vi "Timed motor direction switch.vi"() -> ()   [LabVIEW 2015]
panel:
  out "GREEN = PASS 2":bool caption="Passed"
  out "Sheath Forward":dynamicdata(graph) caption="Tested Signals"
  out "Guide Backward":dynamicdata(graph) caption="Tested Signals"
  out "Guide Forward":dynamicdata(graph) caption="Tested Signals"
  out "XY Graph":cluster{"X":dbl, "Y":dbl}[](graph)
  out "Encoder Graph":waveform(dbl)(graph)
  in  "Sensei":bool
  in  "Boolean 10":bool
  in  "Boolean 9":bool
  in  "Boolean 8":bool
  in  "Boolean 7":bool
  in  "Boolean 6":bool
  in  "Boolean 5":bool
  in  "Boolean 4":bool
  in  "Boolean 3":bool
  out "GREEN = PASS":bool caption="Passed"
  out "Sheath Forward":dynamicdata(graph) caption="Tested Signals"
  out "V v. t (2nd)":cluster{"X":dbl, "Y":dbl}[](graph)
  out "T v. t (2nd)":cluster{"X":dbl, "Y":dbl}[](graph)
  out "V v. t (1st)":cluster{"X":dbl, "Y":dbl}[](graph)
  out "T v. t (1st)":cluster{"X":dbl, "Y":dbl}[](graph)
  in  "TORQUE SET POINT":dbl caption="Torque setpoint"
  # "SELECT MOTOR AND PRESS RUN"
  # "SELECT ONE MOTOR AT A TIME"
  # "Guide Carriage"
  # "Sheath Carriage"
  # "Magellan"
  # "3\n7"
  # "X\n2"
  # "6\n3"
  # "2\n8"
  # "X\n1"
  # "4\n9"
  # "7\n4"
  # "1\n6"
  # "FORWARD ROTATION"
  # "BACKWARD ROTATION"
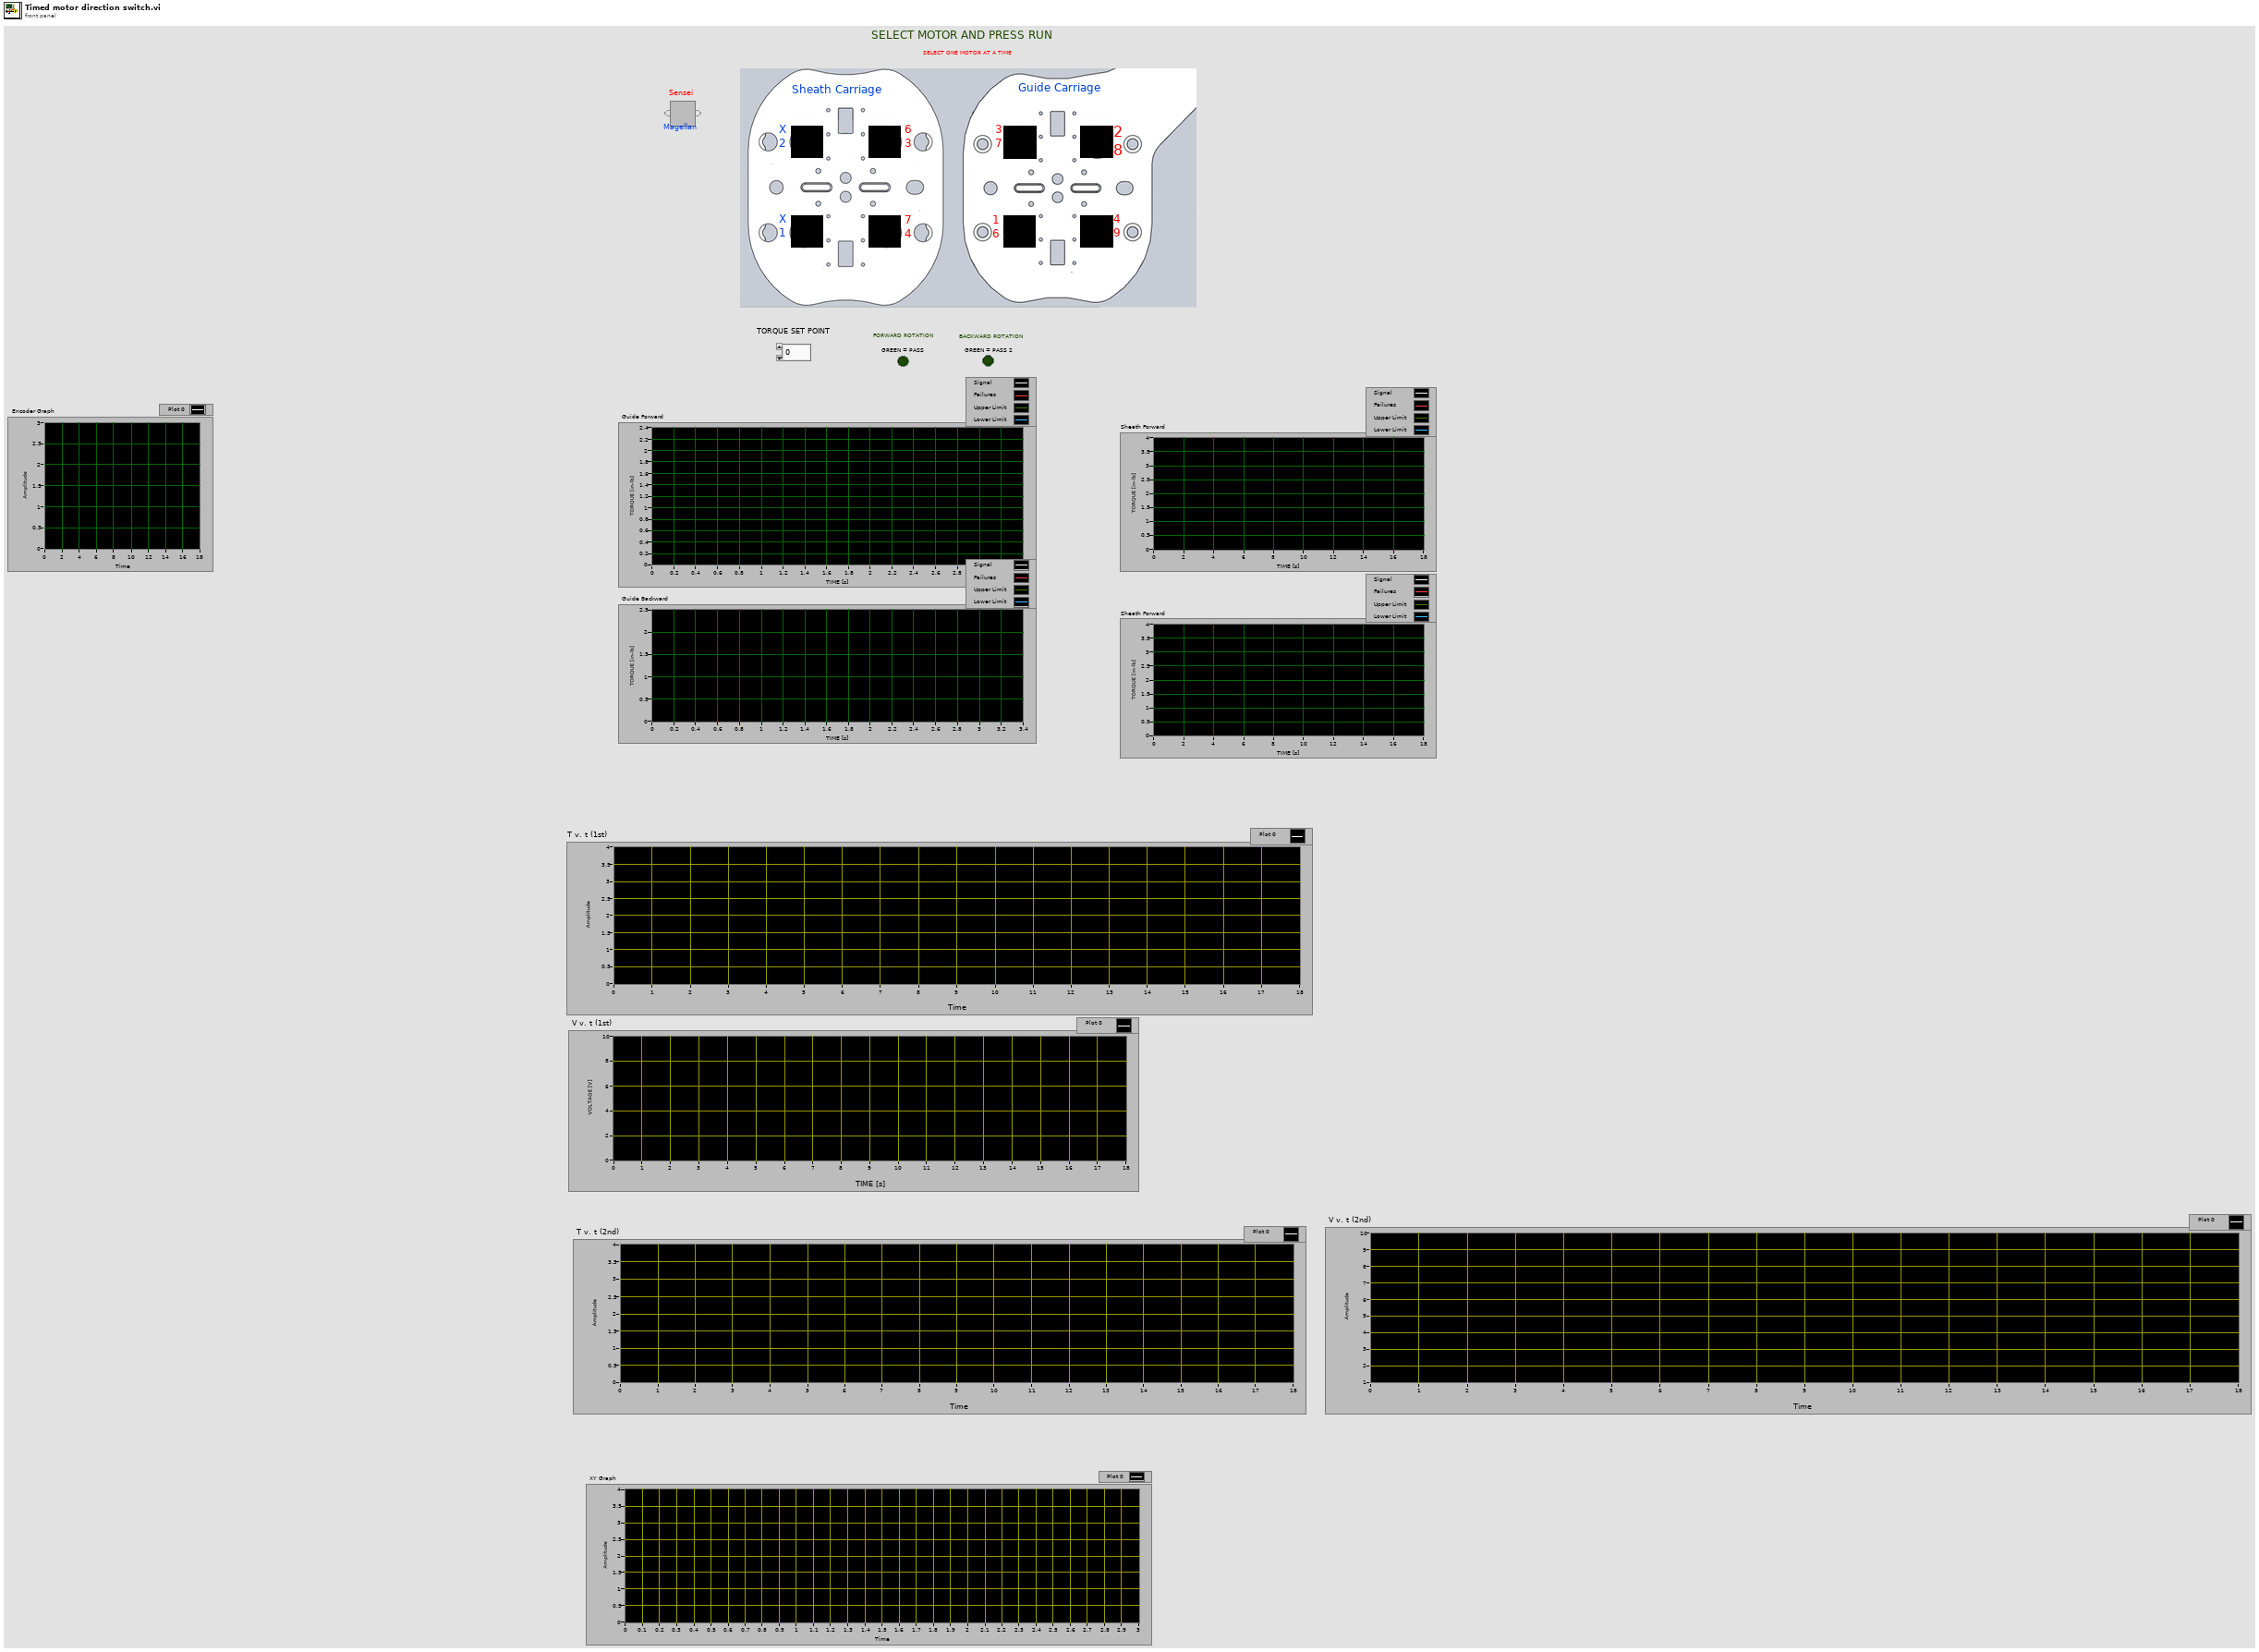
[diagram p1: front panel]
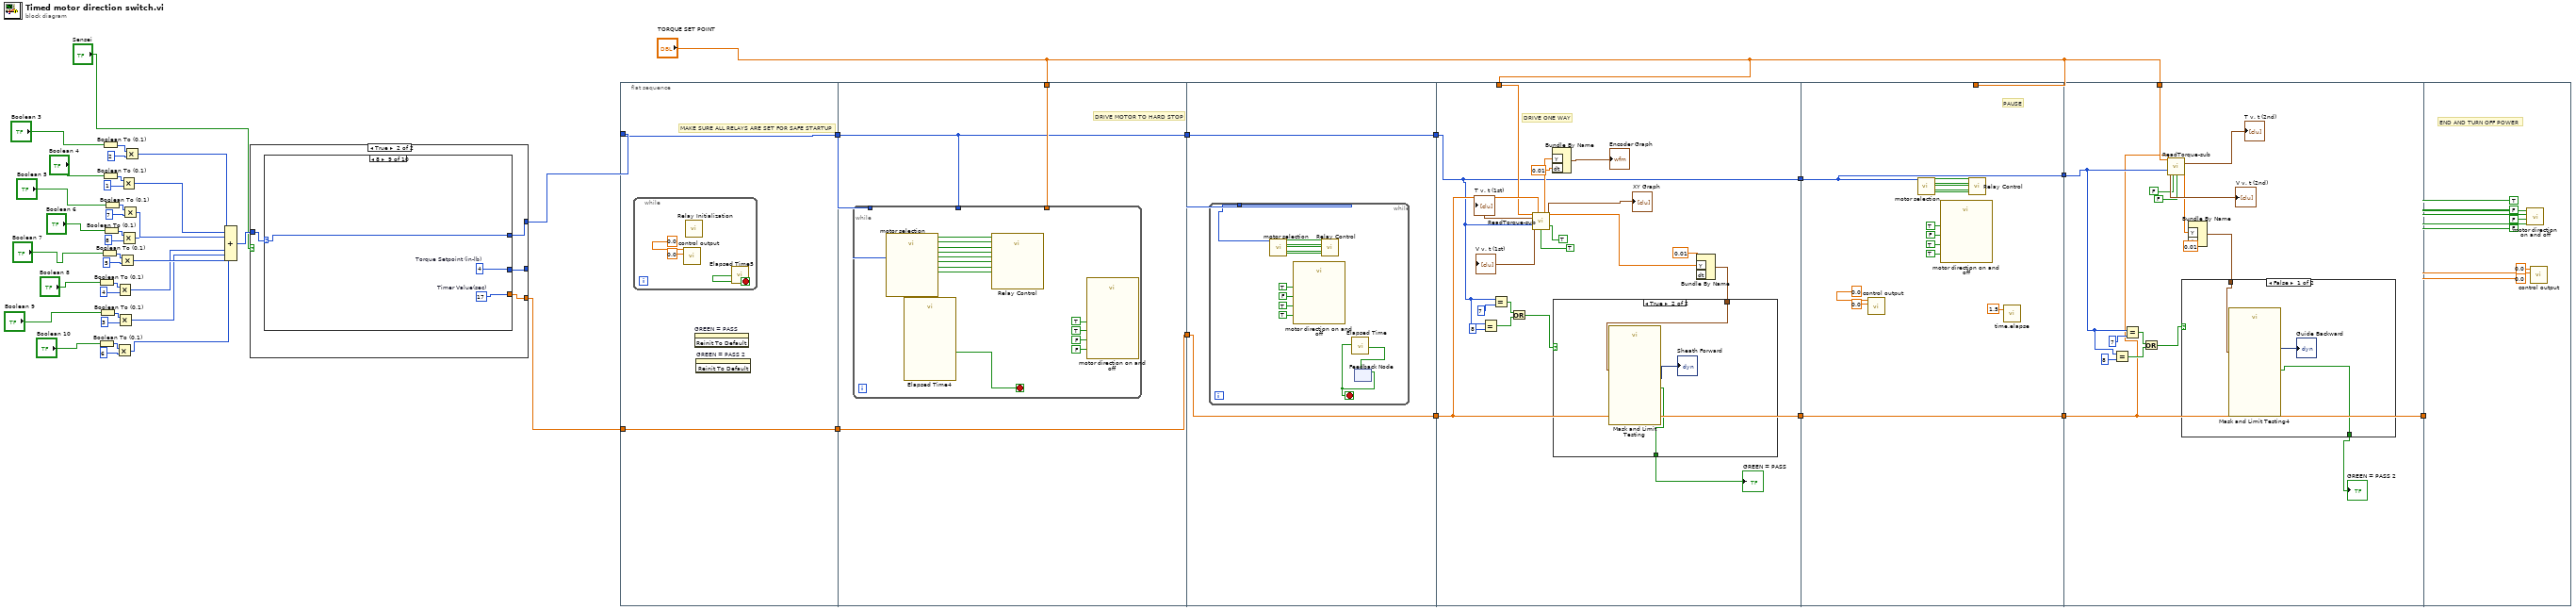
[diagram p0: block diagram]
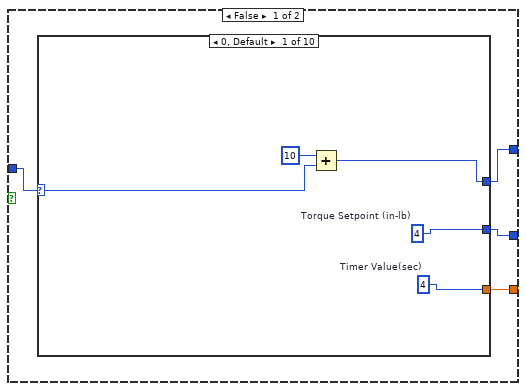
[diagram p2: hidden frame]
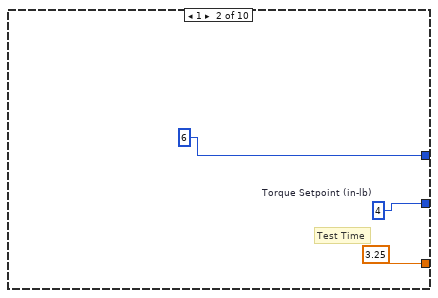
[diagram p3: hidden frame]
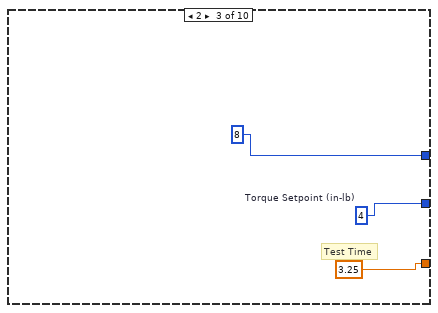
[diagram p4: hidden frame]
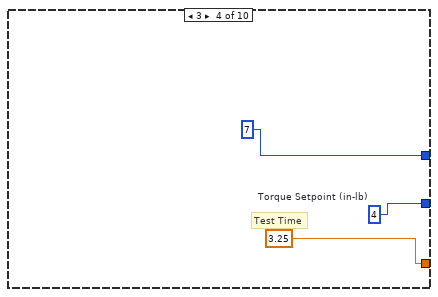
[diagram p5: hidden frame]
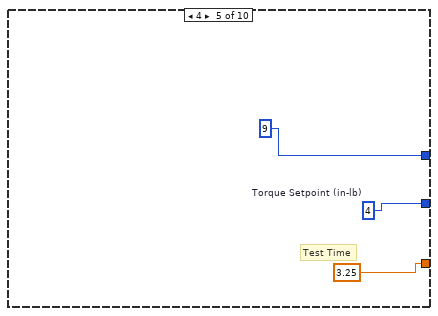
[diagram p6: hidden frame]
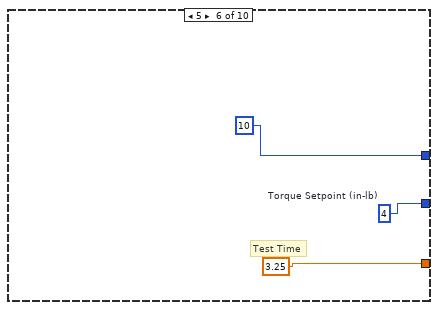
[diagram p7: hidden frame]
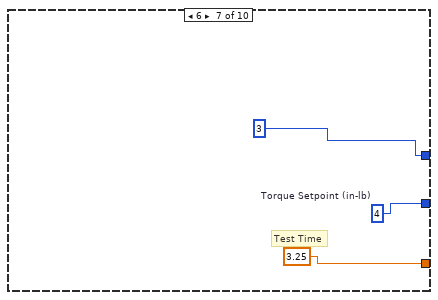
[diagram p8: hidden frame]
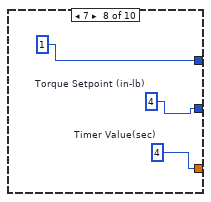
[diagram p9: hidden frame]
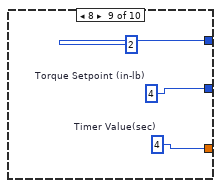
[diagram p10: hidden frame]
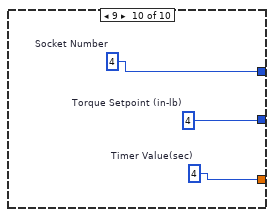
[diagram p11: hidden frame]
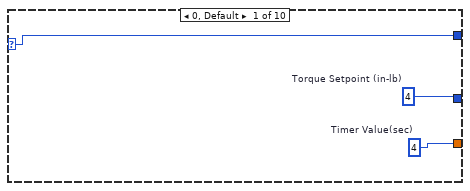
[diagram p12: hidden frame]
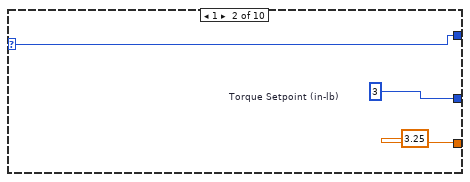
[diagram p13: hidden frame]
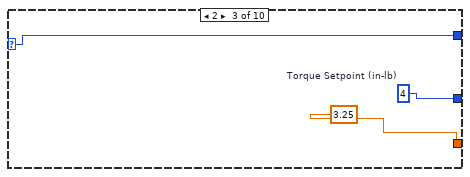
[diagram p14: hidden frame]
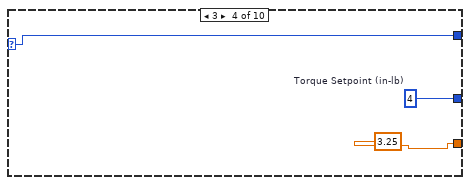
[diagram p15: hidden frame]
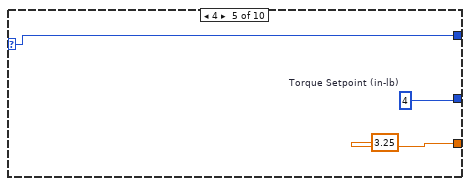
[diagram p16: hidden frame]
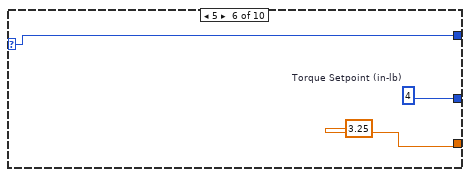
[diagram p17: hidden frame]
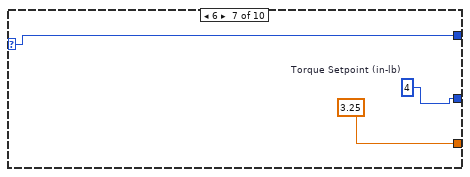
[diagram p18: hidden frame]
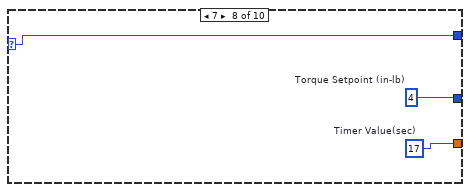
[diagram p19: hidden frame]
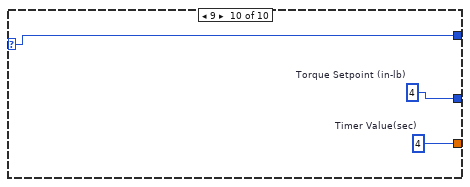
[diagram p20: hidden frame]
diagram:
  n1 = Boolean To (0,1)(Boolean="Boolean 10") -> (0, 1=w28:i16)
  n2 = Boolean To (0,1)(Boolean="Boolean 8") -> (0, 1=w32:i16)
  n3 = Boolean To (0,1)(Boolean="Boolean 9") -> (0, 1=w30:i16)
  n4 = Boolean To (0,1)(Boolean="Boolean 7") -> (0, 1=w34:i16)
  n5 = Boolean To (0,1)(Boolean="Boolean 3") -> (0, 1=w42:i16)
  n6 = Boolean To (0,1)(Boolean="Boolean 4") -> (0, 1=w40:i16)
  n7 = Boolean To (0,1)(Boolean="Boolean 6") -> (0, 1=w36:i16)
  n8 = Boolean To (0,1)(Boolean="Boolean 5") -> (0, 1=w38:i16)
  n9 = Multiply(x=w28, y=i16 6) -> (x*y=w19:i16)
  n10 = Multiply(x=w32, y=i16 4) -> (x*y=w21:i16)
  n11 = Multiply(x=w30, y=i16 3) -> (x*y=w20:i16)
  n12 = Multiply(x=w34, y=i16 5) -> (x*y=w22:i16)
  n13 = Multiply(x=w40, y=i16 1) -> (x*y=w25:i16)
  n14 = Multiply(x=w36, y=i16 8) -> (x*y=w23:i16)
  n15 = Multiply(x=w38, y=i16 7) -> (x*y=w24:i16)
  n16 = Multiply(x=w42, y=i16 2) -> (x*y=w26:i16)
  n17 = Compound Arithmetic op=ADD(w26, w25, w24, w23, w22, w21, w20, w19) -> (w18:i16)
  n18 = case shown="True" "Sensei" {
    tunnel: [w52 w88] -> w8
    tunnel: w18 -> [w51 w87]
    tunnel: [w50 w85] -> w6
    tunnel: [w49 w86] -> _
    frame False {
      n19 = case shown="0, Default" w51 {
        selector: w51 -> [w55 _ _ _ _ _ _ _ _ _]
        tunnel: [w56 6 ("x") 8 ("x") 7 ("x") 9 ("x") 10 ("x") 3 ("x") 1 ("x") 2 ("x") w84] -> w52
        tunnel: [w54 w59 w62 w65 w68 w71 w74 w77 w80 w83] -> w49
        tunnel: [w53 3.25 3.25 3.25 3.25 3.25 3.25 w76 w79 w82] -> w50
        frame 0, Default {
          w53 = 4  # Timer Value(sec)
          w54 = 4  # Torque Setpoint (in-lb)
          n20 = Add(x=10, y=w55) -> (x+y=w56:i32)
        }
        frame 1 {
          w59 = 4  # Torque Setpoint (in-lb)
          # "Test Time"
        }
        frame 2 {
          w62 = 4  # Torque Setpoint (in-lb)
          # "Test Time"
        }
        frame 3 {
          w65 = 4  # Torque Setpoint (in-lb)
          # "Test Time"
        }
        frame 4 {
          w68 = 4  # Torque Setpoint (in-lb)
          # "Test Time"
        }
        frame 5 {
          w71 = 4  # Torque Setpoint (in-lb)
          # "Test Time"
        }
        frame 6 {
          w74 = 4  # Torque Setpoint (in-lb)
          # "Test Time"
        }
        frame 7 {
          w76 = 4  # Timer Value(sec)
          w77 = 4  # Torque Setpoint (in-lb)
        }
        frame 8 {
          w79 = 4  # Timer Value(sec)
          w80 = 4  # Torque Setpoint (in-lb)
        }
        frame 9 {
          w82 = 4  # Timer Value(sec)
          w83 = 4  # Torque Setpoint (in-lb)
          w84 = 4  # Socket Number
        }
      }
    }
    frame True {
      n21 = case shown="8" w87 {
        selector: w87 -> [w91 w94 w97 w100 w103 w106 w109 w112 w115 w118]
        tunnel: [w91 w94 w97 w100 w103 w106 w109 w112 w115 w118] -> w88
        tunnel: [w90 w93 w96 w99 w102 w105 w108 w111 w114 w117] -> w86
        tunnel: [w89 3.25 3.25 3.25 3.25 3.25 3.25 w110 w113 w116] -> w85
        frame 0, Default {
          w89 = 4  # Timer Value(sec)
          w90 = 4  # Torque Setpoint (in-lb)
        }
        frame 1 {
          w93 = 3  # Torque Setpoint (in-lb)
        }
        frame 2 {
          w96 = 4  # Torque Setpoint (in-lb)
        }
        frame 3 {
          w99 = 4  # Torque Setpoint (in-lb)
        }
        frame 4 {
          w102 = 4  # Torque Setpoint (in-lb)
        }
        frame 5 {
          w105 = 4  # Torque Setpoint (in-lb)
        }
        frame 6 {
          w108 = 4  # Torque Setpoint (in-lb)
        }
        frame 7 {
          w110 = 17  # Timer Value(sec)
          w111 = 4  # Torque Setpoint (in-lb)
        }
        frame 8 {
          w113 = 17  # Timer Value(sec)
          w114 = 4  # Torque Setpoint (in-lb)
        }
        frame 9 {
          w116 = 4  # Timer Value(sec)
          w117 = 4  # Torque Setpoint (in-lb)
        }
      }
    }
  }
  n22 = flat-sequence {
    tunnel: w8 -> [w120]
    tunnel: [w120] -> w48
    tunnel: w6 -> [w119]
    tunnel: [w119] -> w5
    tunnel: w48 -> [w125]
    tunnel: [w125] -> w47
    tunnel: "TORQUE SET POINT" -> [w126]
    tunnel: [w124] -> w7
    tunnel: w5 -> [w124]
    tunnel: w47 -> [w142]
    tunnel: [w142] -> w46
    tunnel: w7 -> [w141]
    tunnel: [w141] -> w1
    tunnel: "TORQUE SET POINT" -> [w170]
    tunnel: w46 -> [w164]
    tunnel: [w164] -> w45
    tunnel: [w171] -> w2
    tunnel: w1 -> [w171]
    tunnel: "TORQUE SET POINT" -> [_]
    tunnel: w45 -> [w187]
    tunnel: [w187] -> w44
    tunnel: [w184] -> w3
    tunnel: w2 -> [w184]
    tunnel: "TORQUE SET POINT" -> [w212]
    tunnel: w44 -> [w205]
    tunnel: [w201] -> w4
    tunnel: w3 -> [w201]
    tunnel: w4 -> [_]
    frame #0 {
      # "MAKE SURE ALL RELAYS ARE SET FOR SAFE STARTUP"
      n23 = while {
        stop <- w123 stop-if-true
        n24 = call "control output.vi"("DACB"=0.0, "DACA"=0.0) -> ()  [unwired: 10 in]
        n25 = call "Relay Initialization.vi"() -> ()  [unwired: 12 in]
        n26 = call "Elapsed Time5"() -> ("Time has Elapsed"=w123:bool)  [unwired: 12 in, 7 out]
      }
      n27 = invoke on="GREEN = PASS" class="Bool (strict)" method="Reinit To Default"() -> ()  [unwired: 3 in, 3 out]
      n28 = invoke on="GREEN = PASS 2" class="Bool (strict)" method="Reinit To Default"() -> ()  [unwired: 3 in, 3 out]
    }
    frame #1 {
      # "DRIVE MOTOR TO HARD STOP"
      n29 = while {
        tunnel: w125 -> [w128]
        tunnel: w126 -> [_]
        tunnel: w125 -> [_]
        stop <- w127 stop-if-true
        n30 = call "motor selection.vi"("index 2"=w128) -> ("[0]"=w136:bool, "[1]"=w135:bool, "[2]"=w134:bool, "[3]"=w133:bool, "[4]"=w132:bool, "[5]"=w131:bool, "[6]"=w130:bool, "[7]"=w129:bool)  [unwired: 19 in]
        n31 = call "Elapsed Time4"() -> ("Time has Elapsed"=w127:bool)  [unwired: 12 in, 7 out]
        n32 = call "Relay Control.vi"("State 8"=w136, "State 9"=w135, "State 10"=w134, "State 11"=w133, "State 12"=w132, "State 13"=w131, "State 14"=w130, "State 15"=w129) -> ()  [unwired: 20 in]
        n33 = call "motor direction on and off.vi"("State 3"=FALSE, "State 2"=FALSE, "State 1"=TRUE, "State 0"=TRUE) -> ()  [unwired: 8 in]
      }
    }
    frame #2 {
      n34 = while {
        tunnel: w142 -> [w145]
        stop <- w143 stop-if-true
        n35 = call "motor selection.vi"("index 2"=w145) -> ("[0]"=w157:bool, "[1]"=w156:bool, "[2]"=w155:bool, "[3]"=w154:bool, "[4]"=w153:bool, "[5]"=w152:bool, "[6]"=w151:bool, "[7]"=w150:bool)  [unwired: 19 in]
        n36 = call "motor direction on and off.vi"("State 3"=TRUE, "State 2"=TRUE, "State 1"=FALSE, "State 0"=TRUE) -> ()  [unwired: 8 in]
        n37 = call "Relay Control.vi"("State 8"=w157, "State 9"=w156, "State 10"=w155, "State 11"=w154, "State 12"=w153, "State 13"=w152, "State 14"=w151, "State 15"=w150) -> ()  [unwired: 20 in]
        n38 = feedback #1() -> (w143:bool)  [unwired: 1 in]
        n39 = call "Elapsed Time"("Reset"=w143) -> ("Time has Elapsed"=w144:bool)  [unwired: 11 in, 7 out]
        n40 = feedback-in #1(w144) -> ()
      }
    }
    frame #3 {
      # "DRIVE ONE WAY"
      n41 = Equal?(x=w164, y=8) -> (x = y?=w160:bool)
      n42 = Equal?(x=w164, y=7) -> (x = y?=w161:bool)
      n43 = Or(x=w161, y=w160) -> (x .or. y?=w159:bool)
      n44 = call "ReadTorque-sub.vi"("Torque Setpoint"=w170, "Test Time"=w171, "index 2"=w164, "State 2"=TRUE, "State 3"=TRUE) -> ("Encoder"=w169:dbl[], 4:"Torque"=w173:dbl[], 5:"Torque"=→"T v. t (1st)":cluster{dbl, dbl}[], "Torque vs. Angle"=→"XY Graph":cluster{dbl, dbl}[], "Voltage"=→"V v. t (1st)":cluster{dbl, "voltage out":dbl}[])  [unwired: 3 in, 3 out]
      n45 = Bundle By Name("Y"=w169, "dt"=0.01) -> (→"Encoder Graph":waveform(dbl))  [unwired: 1 in]
      n46 = Bundle By Name("Y"=w173, "dt"=0.01) -> (w165:waveform(dbl))  [unwired: 1 in]
      n47 = case shown="True" w159 {
        tunnel: w165 -> [w179 w182]
        tunnel: [w178 w181] -> w158
        frame False {
          n48 = call "Mask and Limit Testing3"("Signals"=w179) -> ("Passed"=w178:bool, "Tested Signals"=→"Guide Forward":dynamicdata)  [unwired: 7 in, 2 out]
        }
        frame True {
          n49 = call "Mask and Limit Testing"("Signals"=w182) -> ("Passed"=w181:bool, "Tested Signals"=→"Sheath Forward":dynamicdata)  [unwired: 7 in, 2 out]
        }
      }
      "GREEN = PASS" <- w158
    }
    frame #4 {
      # "PAUSE"
      n50 = call "control output.vi"("DACB"=0.0, "DACA"=0.0) -> ()  [unwired: 10 in]
      n51 = call "motor selection.vi"("index 2"=w187) -> ("[0]"=w200:bool, "[1]"=w199:bool, "[2]"=w198:bool, "[3]"=w197:bool, "[4]"=w196:bool, "[5]"=w195:bool, "[6]"=w194:bool, "[7]"=w193:bool)  [unwired: 19 in]
      n52 = call "motor direction on and off.vi"("State 3"=TRUE, "State 2"=TRUE, "State 1"=FALSE, "State 0"=TRUE) -> ()  [unwired: 8 in]
      n53 = call "Relay Control.vi"("State 8"=w200, "State 9"=w199, "State 10"=w198, "State 11"=w197, "State 12"=w196, "State 13"=w195, "State 14"=w194, "State 15"=w193) -> ()  [unwired: 20 in]
      n54 = call "time.elapse.vi"("Set Time"=1.5) -> ()  [unwired: 3 in]
    }
    frame #5 {
      n55 = Equal?(x=w205, y=8) -> (x = y?=w206:bool)
      n56 = Equal?(x=w205, y=7) -> (x = y?=w207:bool)
      n57 = Or(x=w207, y=w206) -> (x .or. y?=w204:bool)
      n58 = call "ReadTorque-sub.vi"("Torque Setpoint"=w212, "Test Time"=w201, "index 2"=w205, "State 2"=FALSE, "State 3"=FALSE) -> (4:"Torque"=w210:dbl[], 5:"Torque"=→"T v. t (2nd)":cluster{dbl, dbl}[], "Voltage"=→"V v. t (2nd)":cluster{dbl, "voltage out":dbl}[])  [unwired: 3 in, 5 out]
      n59 = Bundle By Name("Y"=w210, "dt"=0.01) -> (w203:waveform(dbl))  [unwired: 1 in]
      n60 = case shown="False" w204 {
        tunnel: w203 -> [w218 w221]
        tunnel: [w217 w220] -> w202
        frame False {
          n61 = call "Mask and Limit Testing4"("Signals"=w218) -> ("Passed"=w217:bool, "Tested Signals"=→"Guide Backward":dynamicdata)  [unwired: 7 in, 2 out]
        }
        frame True {
          n62 = call "Mask and Limit Testing2"("Signals"=w221) -> ("Passed"=w220:bool, "Tested Signals"=→"Sheath Forward":dynamicdata)  [unwired: 7 in, 2 out]
        }
      }
      "GREEN = PASS 2" <- w202
    }
    frame #6 {
      # "END AND TURN OFF POWER"
      n63 = call "motor direction on and off.vi"("State 3"=FALSE, "State 2"=FALSE, "State 1"=FALSE, "State 0"=TRUE) -> ()  [unwired: 8 in]
      n64 = call "control output.vi"("DACB"=0.0, "DACA"=0.0) -> ()  [unwired: 10 in]
    }
  }
